vi "Update.vi"(8 "error in":errorcluster, 11 "cPAS Subject in":refnum<class "cPAS Subject.lvclass">) -> (0 "error out":errorcluster, 2 "Stop?":bool, 3 "cPAS Subject out":refnum<class "cPAS Subject.lvclass">)   [LabVIEW 2015, in "cPAS Subject.lvclass"]
doc: "Data for the photoacoustic is retrieved via a shared variable 'Data'. The Update VI checks the SV for fresh data. If there is fresh data, then the 'Data' string is unflattened to the proper type (in this case cPAS Data), stuffed into the DVR (the 'Preserve Runtime Class' VI is required to handle the cast in the 'In Place Element Structure') and the observers are notified via a new element in the queue."
uses:
  cPAS Subject.lvclass
  Data/cPAS Data.lvclass
  Reusable/Data/Data.lvclass
  Reusable/Observer/Data Subject.lvclass/Data Subject.ctl
  Reusable/Observer/Accessors/Read Observer Refs.vi
  Reusable/Observer/Accessors/Read DVR.vi
  Reusable/Observer/Data Subject.lvclass
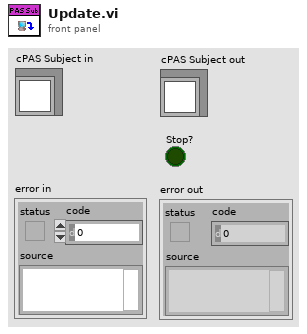
[diagram p1: front panel]
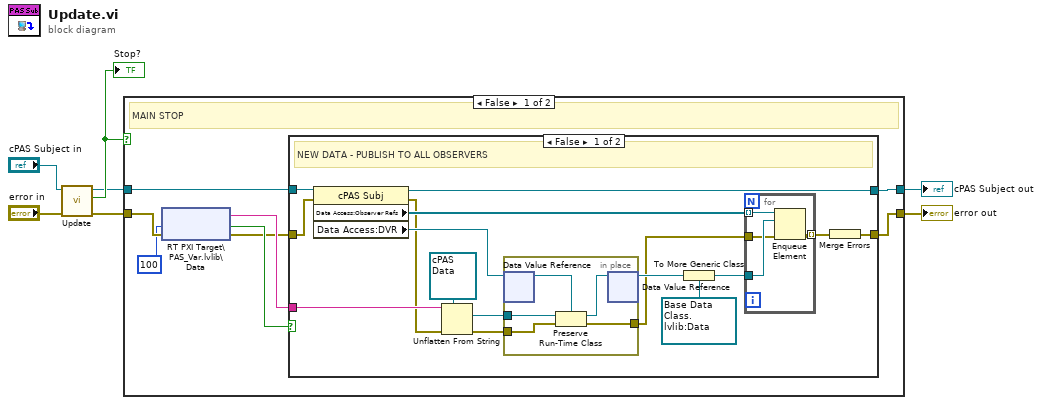
[diagram p0: block diagram]
diagram:
  n1 = call-parent "Update.vi"("error in"="error in", "Data Subject in"="cPAS Subject in") -> ("error out"=w4:errorcluster, "Stop?"=w5:bool, "Data Subject out"=w3:refnum<class "cPAS Subject.lvclass">)  [unwired: 7 in]
  "Stop?" <- w5
  n2 = case shown="False" w5 {
    tunnel: w3 -> [w11 w44]
    tunnel: w4 -> [w15 w43]
    tunnel: [w10 w44] -> w2
    tunnel: [w8 w43] -> w1
    frame False {
      # "MAIN STOP"
      n3 = shared-variable "RT PXI Target\\PAS_Var.lvlib\\Data"(error in=w15, 100 ("ms timeout (0)")) -> (w13:string, error out=w9:errorcluster, w12:bool)
      n4 = case shown="False" w12 {
        tunnel: w13 -> [w27 _]
        tunnel: w11 -> [w26 w42]
        tunnel: [w23 w42] -> w10
        tunnel: w9 -> [w22 w41]
        tunnel: [w16 w41] -> w8
        frame False {
          # "NEW DATA - PUBLISH TO ALL OBSERVERS"
          n5 = property class="cPAS Subj"(reference=w26, error in=w22) -> (reference out=w23:refnum<class "cPAS Subject.lvclass">, error out=w20:errorcluster, "Data Access:Observer Refs"=w25:refnum<queue>[], "Data Access:DVR"=w24:refnum<data-value>)
          n6 = Unflatten From String(type=refnum<class "cPAS Data.lvclass"> refnum ("cPAS Data"), binary string=w27, error in (no error)=w20) -> (value=w28:refnum<class "cPAS Data.lvclass">, error out=w19:errorcluster)  [unwired: 2 in, 1 out]
          n7 = in-place {
            in-place-border: w28 -> [w40]
            in-place-border: [w37] -> w18
            in-place-border: w19 -> [w36]
            n8 = in-place-dvr #1(w24) -> (w39:refnum<class "Data.lvclass">)  [unwired: 1 out]
            n9 = Preserve Run-Time Class(object in=w40, error in=w36, 2:w39) -> (object out=w38:refnum<class "Data.lvclass">, error out=w37:errorcluster)
            n10 = in-place-dvr #1(w38) -> (w30:refnum<data-value>)  [unwired: 1 out]
          }
          n11 = To More Generic Class(target class=refnum<data-value> refnum ("data value reference"), reference=w30) -> (generic class reference=w29:refnum<data-value>)
          n12 = for {
            tunnel: w29 -> [w35]
            tunnel: w25 -> [w34] mode=indexing
            tunnel: w18 -> [w33]
            tunnel: [w32] -> w17 mode=indexing
            n13 = Enqueue Element(queue=w34, element=w35, error in (no error)=w33) -> (error out=w32:errorcluster)  [unwired: 1 in, 2 out]
          }
          n14 = Merge Errors(w17) -> (w16:errorcluster)
        }
        frame True {
          # "NO DATA AVAILABLE"
        }
      }
    }
    frame True {
    }
  }
  "error out" <- w1
  "cPAS Subject out" <- w2
